vi "Restrict X Range (single).vi"(8 "error in (no error)":errorcluster, 9 "X Max":dbl, 10 "X Min":dbl, 11 "XY-data":cluster{"X-array":dbl[], "Y-array":dbl[]}) -> (0 "error out":errorcluster, 3 "XY-data out":cluster{"X-array":dbl[], "Y-array":dbl[]} {"Y-array" format="%.2p"; "X-array" format="%.2p"})   [LabVIEW 2019, in "xy_utilities.lvlib"]
doc: "Removes data points that fall outside of the range defined by <b>X Min</b> and <b>X Max</b>s\n\nWire data to the data input to determine the polymorphic instance to use or manually select the instance."
uses:
  xy_utilities.lvlib
  <vilib>/Analysis/NI_AALPro.lvlib
  <vilib>/Analysis/6fits.llb/Remove Outliers (Range).vi
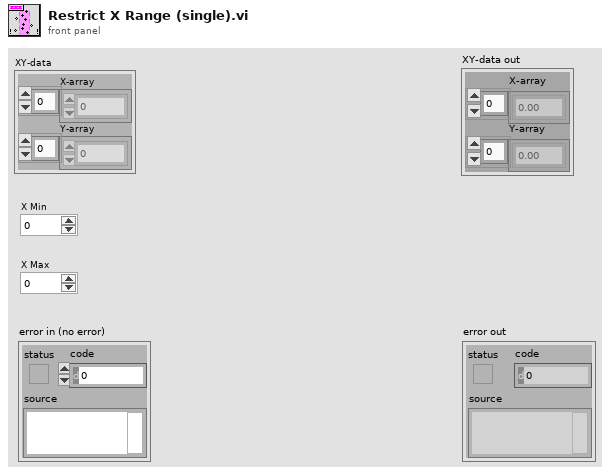
[diagram p1: front panel]
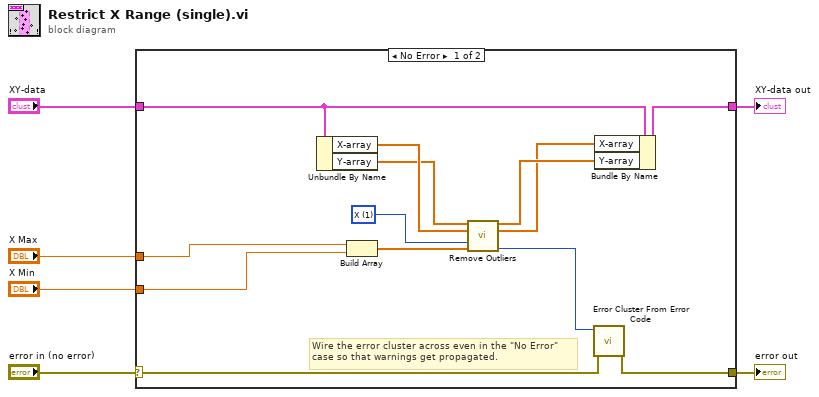
[diagram p0: block diagram]
diagram:
  n1 = case shown="No Error" "error in (no error)" {
    selector: "error in (no error)" -> [w9 w21]
    tunnel: [w8 w21] -> w5
    tunnel: "XY-data" -> [w19 w20]
    tunnel: [w18 w20] -> w3
    tunnel: "X Max" -> [w11 _]
    tunnel: "X Min" -> [w12 _]
    frame No Error {
      w7 = u16 1 items=["Y", "X", "X and Y"] ("range type")
      # "Wire the error cluster across even in the \"No Error\"\ncase so that warnings get propagated."
      n2 = Unbundle By Name(w19) -> ("X-array"=w16:dbl[], "Y-array"=w15:dbl[])
      n3 = Build Array(w11, w12) -> (w17:dbl[])
      n4 = call-poly <vilib>:"Remove Outliers.vi"("Y"=w15, "X"=w16, "range type"=w7, "Range"=w17) -> ("Y Out"=w14:dbl[], "X Out"=w13:dbl[], "error"=w10:i32)  [unwired: 7 in, 2 out]
      n5 = call <vilib>:"Error Cluster From Error Code.vi"("error in (no error)"=w9, "error code (0)"=w10) -> ("error out"=w8:errorcluster)  [unwired: 7 in]
      n6 = Bundle By Name(cluster=w19, "X-array"=w13, "Y-array"=w14) -> (w18:cluster{"X-array":dbl[], "Y-array":dbl[]})
    }
    frame Error {
    }
  }
  "error out" <- w5
  "XY-data out" <- w3
